vi "State Vector Array.vi"(7 "QuWire in":refnum<class "QuWire.lvclass">) -> (4 "State Vector":cdb[](array[numeric]), 15 "Qubits n":i32)   [LabVIEW 2020]
uses:
  QuSim/QuWire/QuWire.lvclass
panel:
  out "Basis States and State Vector":cluster{"State":i32, "Probability":cdb}[](array[cluster]) {"Probability" format="%#.6f"; "State" format="%07b"}
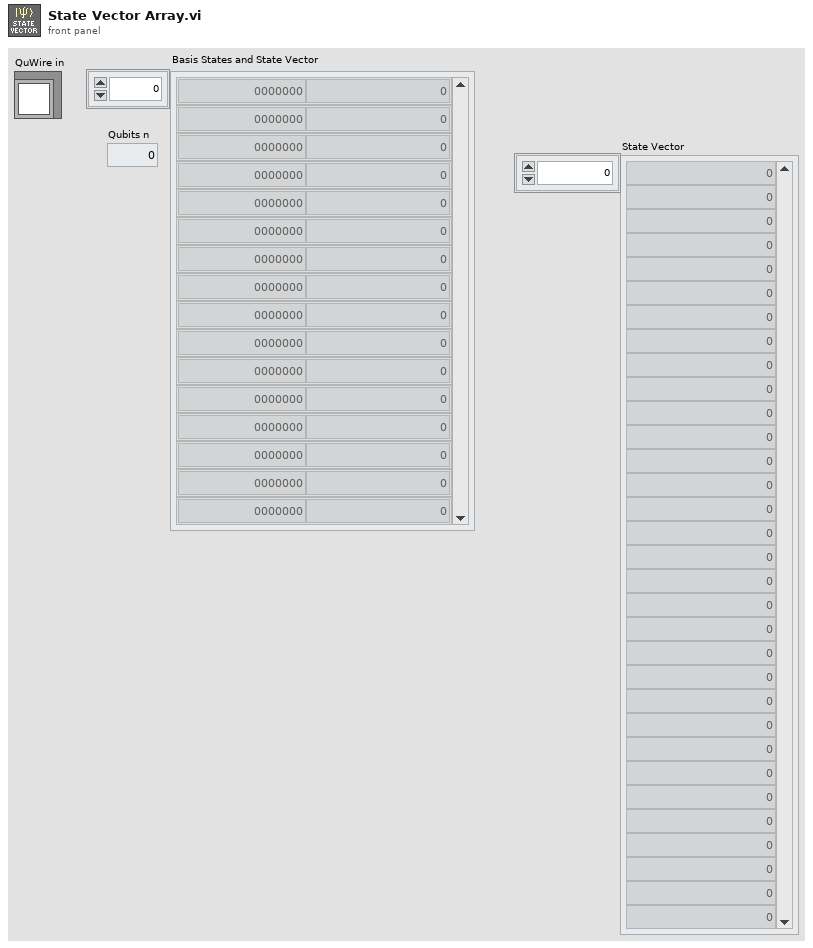
[diagram p1: front panel]
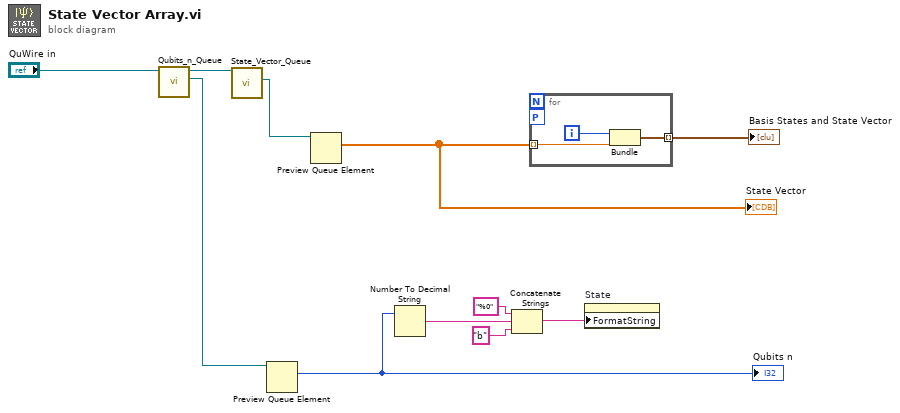
[diagram p0: block diagram]
diagram:
  n1 = call "Qubits_n_Queue.vi"("QuWire in"="QuWire in") -> ("Qubit n"=w3:refnum<queue>, "QuWire out"=w4:refnum<class "QuWire.lvclass">)  [unwired: 8 in, 1 out]
  n2 = call "State_Vector_Queue.vi"("QuWire in"=w4) -> ("State Vector Queue"=w10:refnum<queue>)  [unwired: 8 in, 2 out]
  n3 = Preview Queue Element(queue=w3) -> (element=w8:i32)  [unwired: 2 in, 3 out]
  "Qubits n" <- w8
  n4 = Preview Queue Element(queue=w10) -> (element=w1:cdb[])  [unwired: 2 in, 3 out]
  "State Vector" <- w1
  n5 = Number To Decimal String(number=w8) -> (decimal integer string=w7:string)  [unwired: 1 in]
  n6 = Concatenate Strings("%0" ("string"), w7, "b" ("string")) -> (w2:string)
  n7 = for {
    tunnel: w1 -> [w13] mode=indexing
    tunnel: [w12] -> w9 mode=indexing
    workers-P: _ -> [_]
    i -> [w14]
    n8 = Bundle(w14, "Complex Matrix Element"=w13) -> (w12:cluster{i32, "Complex Matrix Element":cdb})  [unwired: 1 in]
  }
  "Basis States and State Vector" <- w9
  n9 = property on="State" class="DigNum (strict)"("FormatString"=w2) -> ()  [unwired: 2 in, 2 out]
